vi "MouseWheelMoveStage.vi"(0 "Camera_Prime95B in":refnum<class "Camera_Prime95B.lvclass">, 5 "Label":string, 7 "AbsPosition?":bool=TRUE, 9 "Value":dbl format="%#_13g", 11 "error in (no error)":errorcluster) -> (4 "Camera_Prime95B out":refnum<class "Camera_Prime95B.lvclass">, 15 "error out":errorcluster)   [LabVIEW 2020, in "Camera_Prime95B.lvlib" / "Camera_Prime95B.lvclass"]
uses:
  Camera_Prime95B.lvclass
  C:/Program Files/National Instruments/LabVIEW 2020/vi.lib/ActorFramework/Actor/Actor.lvclass
  <vilib>/ActorFramework/Actor/Actor.lvclass/Actor.ctl
  Interface/MicroscopeIO Messages/SetStagePosition Msg/SetStagePosition Msg.lvclass/SetStagePosition Msg.ctl
  <vilib>/ActorFramework/Message Enqueuer/Message Enqueuer.lvclass/Message Enqueuer.ctl
  <vilib>/ActorFramework/Message Enqueuer/Enqueue.vi
  Interface/MicroscopeIO Messages/SetStagePosition Msg/SetStagePosition Msg.lvclass
  C:/Program Files/National Instruments/LabVIEW 2020/vi.lib/ActorFramework/Message/Message.lvclass
  <vilib>/ActorFramework/Message Priority Queue/Priority Enqueue.vi
  <vilib>/ActorFramework/Actor/Actor.lvclass
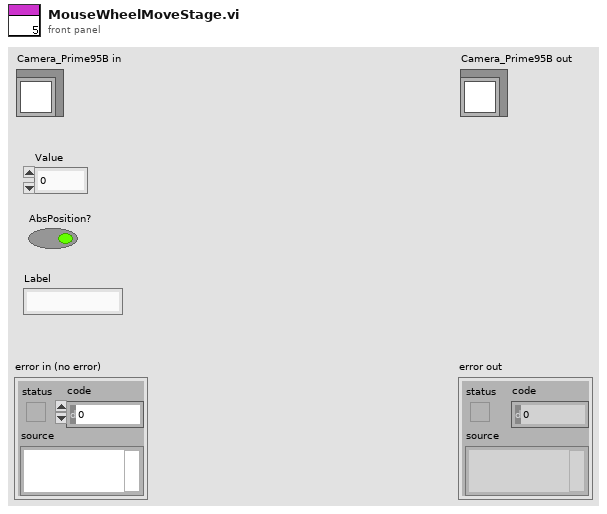
[diagram p1: front panel]
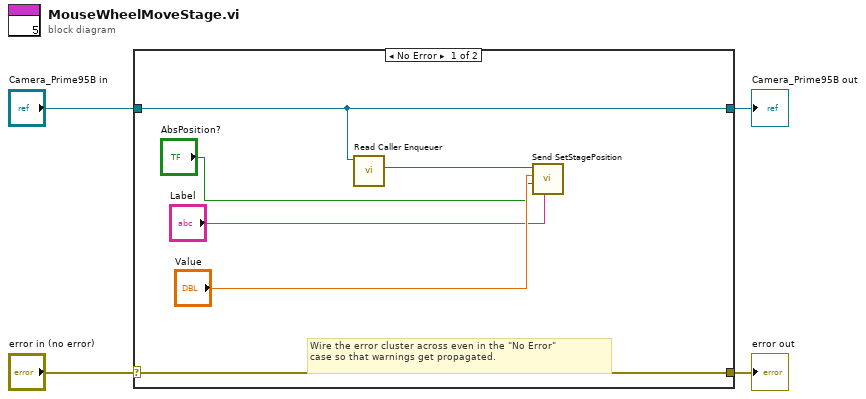
[diagram p0: block diagram]
diagram:
  n1 = case shown="No Error" "error in (no error)" {
    selector: "error in (no error)" -> [w10 w12]
    tunnel: [w10 w12] -> w3
    tunnel: [w9 w11] -> w1
    tunnel: "Camera_Prime95B in" -> [w9 w11]
    frame No Error {
      # "Wire the error cluster across even in the \"No Error\"\ncase so that warnings get propagated."
      n2 = call <vilib>:"Read Caller Enqueuer.vi"("Actor"=w9) -> ("Caller Enqueuer"=w8:refnum<class "Message Enqueuer.lvclass">)  [unwired: 10 in]
      n3 = call "Send SetStagePosition.vi"("Label"="Label", "AbsPosition?"="AbsPosition?", "Value"="Value", "Message Enqueuer"=w8) -> ()  [unwired: 6 in, 2 out]
    }
    frame Error {
    }
  }
  "error out" <- w3
  "Camera_Prime95B out" <- w1
